vi "Single Bscan - DAQ Trigger.vi"(6 "Frequency":cluster{"Clock, kHz":dbl, "Freq, kHz":dbl}={"Clock, kHz"=935.6, "Freq, kHz"=46.78} {"Clock, kHz" format="%#_13g"}, 7 "# Extra":cluster{"# ARpt_extra":i32, "#Brtn_extra":i32}={"# ARpt_extra"=5, "#Brtn_extra"=40}, 9 "Galvo VPP":cluster{"VPP-X":dbl, "VPP-Y":dbl}={"VPP-X"=5.0, "VPP-Y"=5.0}, 10 "Scan Repeat":cluster{"# A rpt":i32, "# B rpt":i32}={"# A rpt"=1, "# B rpt"=1}, 11 "# Points":cluster{"# Aline":i32, "# B scan":i32}={"# Aline"=500, "# B scan"=500}) -> (2 "Galvo X&Trigger":waveform(dbl)[](graph)=[{"t0"=timestamp(0 s since 1904-01-01), "dt"=1.0, "Y"=array[8820 elements]}, {"t0"=timestamp(0 s since 1904-01-01), "dt"=1.0, "Y"=array[8820 elements]}])   [LabVIEW 2017]
uses:
  <vilib>/Waveform/WDTOps.llb/WDT Append Waveforms DBL.vi
  <vilib>/measure/NI_MABase.lvlib
panel:
  out "# A Rpt Delay":i32
  out "# B rtn":i32
  out "# A repeat":i32
  out "dVX":dbl
  out "S/F":dbl
  out "VPP-Y":dbl
  out "VPP-X":dbl
  out "Clock, kHz":dbl
  out "Freq, kHz":dbl
  out "# A Total":i32
  out "# Aline":i32
  out "# B scan":i32
  out "# B Repeat":i32
  # "Single Bscan - DAQ Trigger"
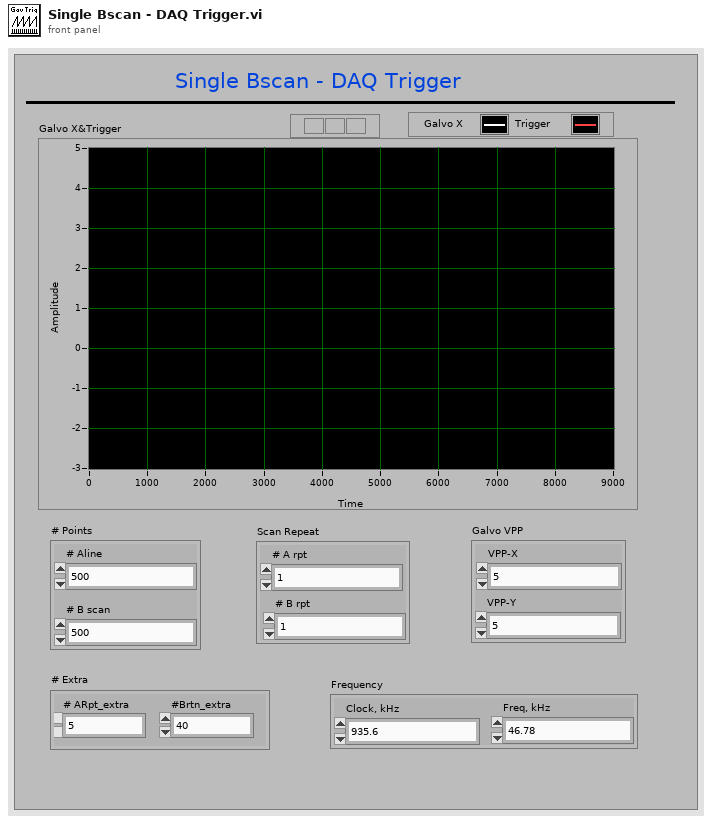
[diagram p1: front panel]
types:
  T1 = enum16{"Sine Wave", "Triangle Wave", "Square Wave", "Sawtooth Wave"}
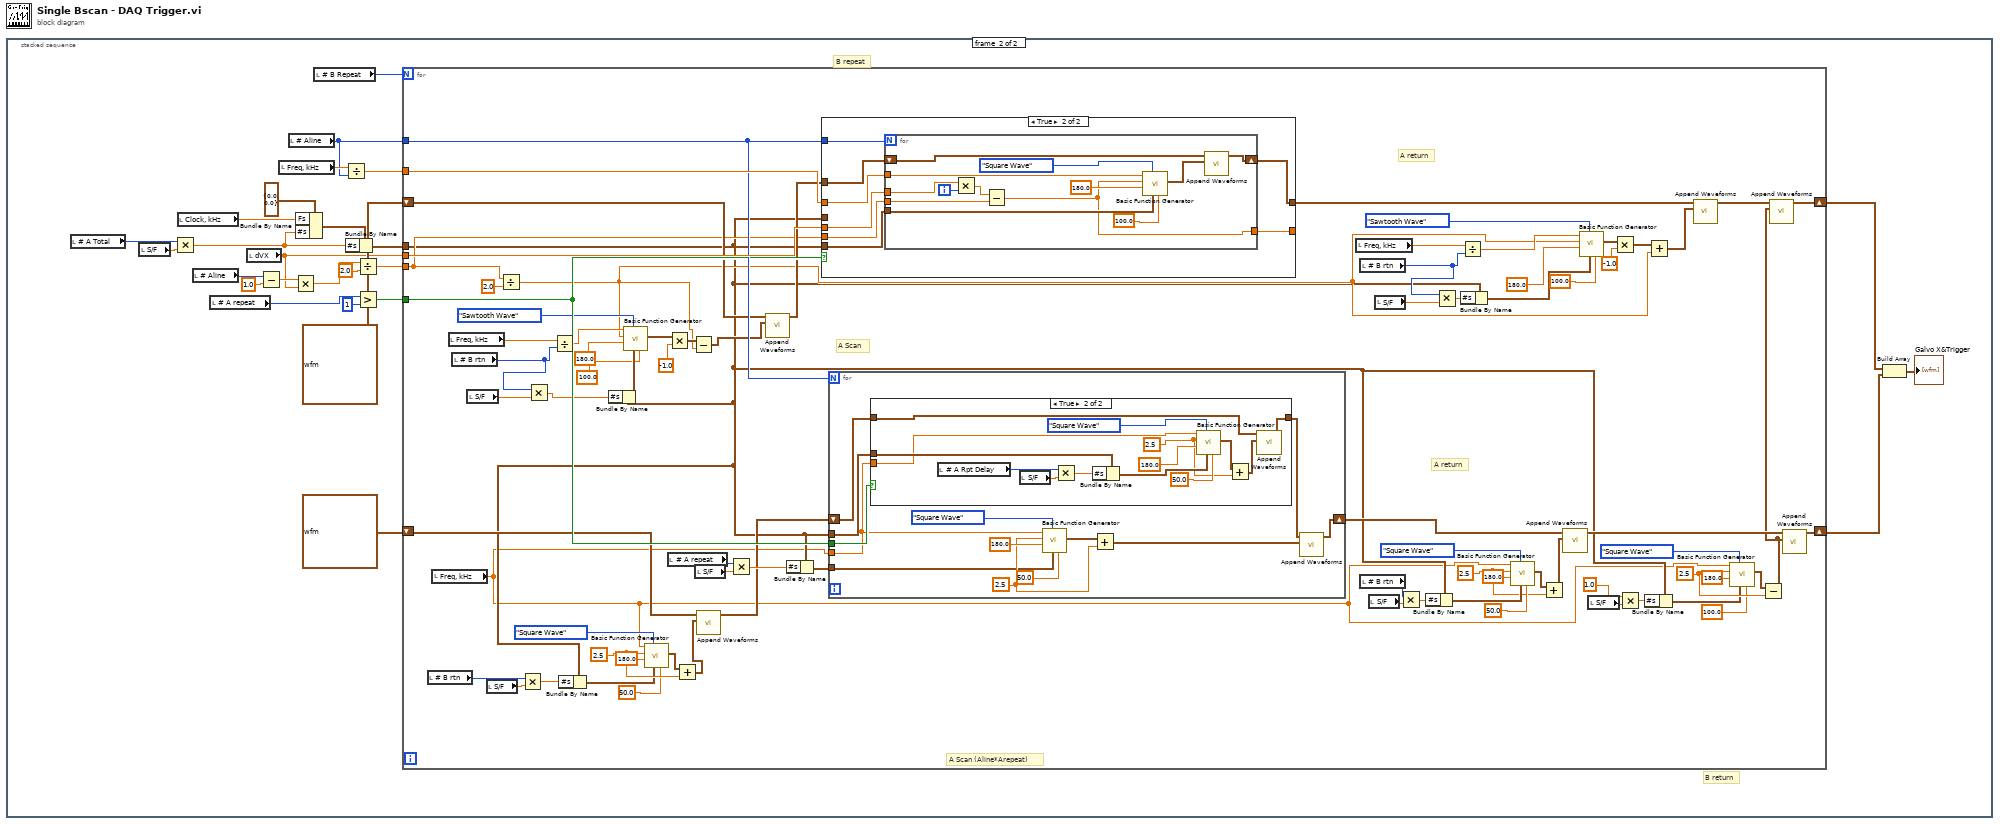
[diagram p0: block diagram]
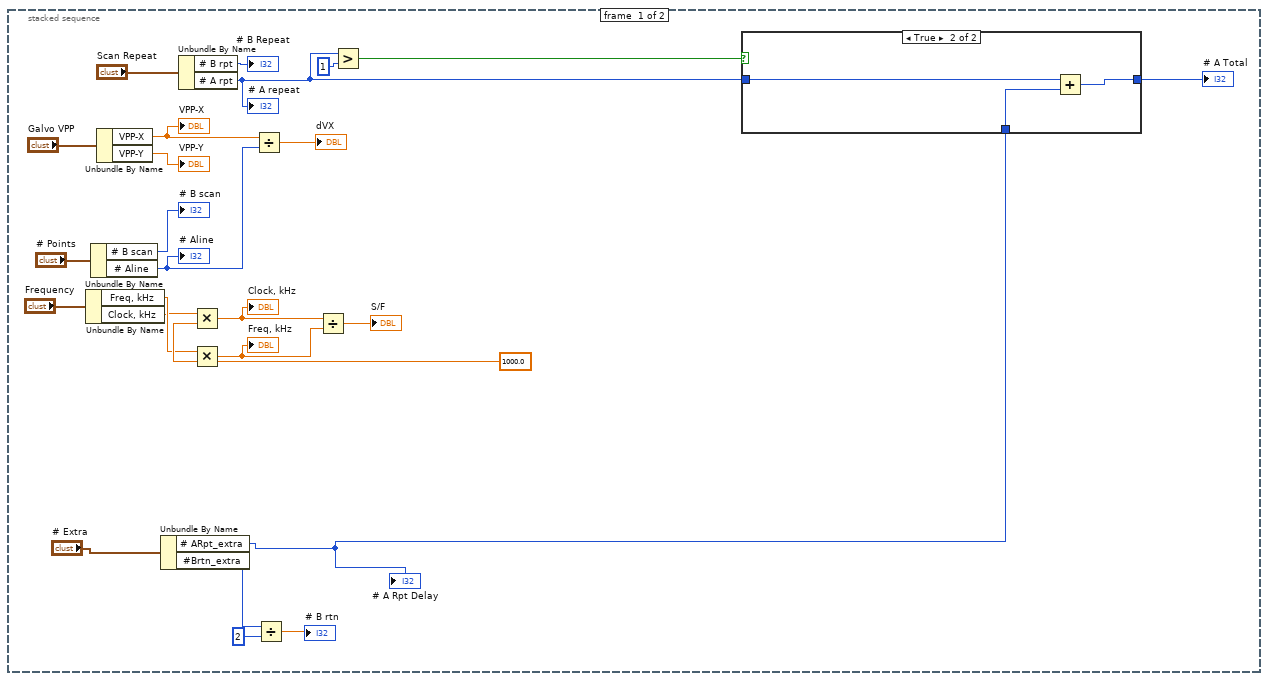
[diagram p2: hidden frame]
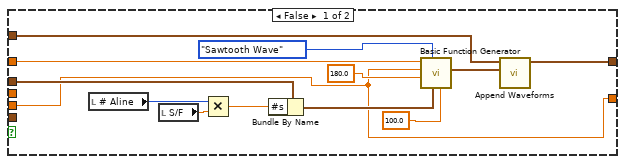
[diagram p5: hidden frame]
diagram:
  n1 = stacked-sequence {
    frame #0 {
      w24 = 1000.0 ("y")
      n2 = Unbundle By Name("Frequency") -> ("Freq, kHz"=w23:dbl, "Clock, kHz"=w19:dbl)
      n3 = Unbundle By Name("# Points") -> ("# B scan"=→"# B scan":i32, "# Aline"=w9:i32)
      "# Aline" <- w9
      n4 = Unbundle By Name("Galvo VPP") -> ("VPP-X"=w8:dbl, "VPP-Y"=→"VPP-Y":dbl)
      "VPP-X" <- w8
      n5 = Unbundle By Name("# Extra") -> ("# ARpt_extra"=w5:i32, "#Brtn_extra"=w4:i32)
      "# A Rpt Delay" <- w5
      n6 = Unbundle By Name("Scan Repeat") -> ("# B rpt"=→"# B Repeat":i32, "# A rpt"=w6:i32)
      "# A repeat" <- w6
      n7 = Multiply(x=w19, y=w24) -> (x*y=w12:dbl)
      "Clock, kHz" <- w12
      n8 = Multiply(x=w23, y=w24) -> (x*y=w11:dbl)
      "Freq, kHz" <- w11
      n9 = Divide(x=w8, y=w9) -> (x/y=→"dVX":dbl)
      n10 = Divide(x=w4, y=2) -> (x/y=→"# B rtn":dbl)
      n11 = Divide(x=w12, y=w11) -> (x/y=→"S/F":dbl)
      n12 = Greater?(x=w6, y=1) -> (0:w20:bool)
      n13 = case shown="True" w20 {
        tunnel: w6 -> [w26 w29]
        tunnel: [w26 w28] -> w22
        tunnel: w5 -> [_ w27]
        frame False {
        }
        frame True {
          n14 = Add(x=w29, y=w27) -> (x+y=w28:i32)
        }
      }
      "# A Total" <- w22
    }
    frame #1 {
      # "B return"
      # "B repeat"
      n15 = local read "# A Total"() -> (w42:i32)
      n16 = local read "S/F"() -> (w41:dbl)
      n17 = Multiply(x=w42, y=w41) -> (x*y=w40:dbl)
      n18 = local read "Clock, kHz"() -> (w43:dbl)
      n19 = local read "# Aline"() -> (w44:i32)
      n20 = local read "# A repeat"() -> (w39:i32)
      n21 = local read "dVX"() -> (w33:dbl)
      n22 = Subtract(x=w44, y=1.0) -> (x-y=w46:dbl)
      n23 = local read "Freq, kHz"() -> (w36:dbl)
      n24 = local read "# Aline"() -> (w35:i32)
      n25 = Multiply(x=w46, y=w33) -> (x*y=w50:dbl)
      n26 = Bundle By Name(cluster=cluster{"Fs":dbl, "#s":dbl} {"Fs"=0.0, "#s"=0.0} ("input cluster"), "Fs"=w43, "#s"=w40) -> (w51:cluster{"Fs":dbl, "#s":dbl})
      n27 = local read "# B Repeat"() -> (w45:i32)
      n28 = Divide(x=w36, y=w35) -> (x/y=w34:dbl)
      n29 = Bundle By Name(cluster=w51, "#s"=w40) -> (w53:cluster{"Fs":dbl, "#s":dbl})
      n30 = Divide(x=w50, y=2.0) -> (x/y=w48:dbl)
      n31 = Greater?(x=w39, y=1) -> (0:w37:bool)
      n32 = for {
        N: w45 -> [_]
        tunnel: w35 -> [w110]
        tunnel: w33 -> [w134]
        tunnel: w53 -> [w61]
        tunnel: w48 -> [w94]
        shift-right: [w58] -> w30
        shift-left: waveform(dbl) {"t0"=timestamp(0 s since 1904-01-01), "dt"=1.0, "Y"=[]} ("waveform out") -> [w98]
        tunnel: w37 -> [w109]
        tunnel: w34 -> [w133]
        shift-right: [w62] -> w31
        shift-left: waveform(dbl) {"t0"=timestamp(0 s since 1904-01-01), "dt"=1.0, "Y"=[]} ("waveform out") -> [w75]
        w70 = 2.5 ("amplitude")
        w84 = 2.5 ("amplitude")
        w85 = 2.5 ("amplitude")
        # "A Scan"
        # "A return"
        # "A Scan (Aline*Arepeat)"
        # "A return"
        n33 = local read "# B rtn"() -> (w79:i32)
        n34 = local read "Freq, kHz"() -> (w60:dbl)
        n35 = local read "Freq, kHz"() -> (w104:dbl)
        n36 = local read "# B rtn"() -> (w107:i32)
        n37 = local read "S/F"() -> (w103:dbl)
        n38 = local read "S/F"() -> (w80:dbl)
        n39 = Divide(x=w94, y=2.0) -> (x/y=w88:dbl)
        n40 = Multiply(x=w79, y=w80) -> (x*y=w81:dbl)
        n41 = Multiply(x=w107, y=w103) -> (x*y=w106:dbl)
        n42 = Divide(x=w104, y=w107) -> (x/y=w105:dbl)
        n43 = Bundle By Name(cluster=w61, "#s"=w81) -> (w76:cluster{"Fs":dbl, "#s":dbl})
        n44 = Bundle By Name(cluster=w61, "#s"=w106) -> (w102:cluster{"Fs":dbl, "#s":dbl})
        n45 = call <vilib>:"Basic Function Generator.vi"("square wave duty cycle (%)"=100.0, "sampling info"=w102, "signal type"=T1."Sawtooth Wave", "phase"=180.0, "amplitude"=w88, "frequency"=w105) -> ("signal out"=w96:waveform(dbl))  [unwired: 3 in, 2 out]
        n46 = call <vilib>:"Basic Function Generator.vi"("square wave duty cycle (%)"=50.0, "sampling info"=w76, "signal type"=T1."Square Wave", "phase"=180.0, "amplitude"=w84, "frequency"=w60) -> ("signal out"=w82:waveform(dbl))  [unwired: 3 in, 2 out]
        n47 = Multiply(x=w96, y=-1.0) -> (x*y=w92:waveform(dbl))
        n48 = local read "# A repeat"() -> (w116:i32)
        n49 = Add(x=w82, y=w84) -> (x+y=w83:waveform(dbl))
        n50 = Subtract(x=w92, y=w88) -> (x-y=w91:waveform(dbl))
        n51 = local read "S/F"() -> (w114:dbl)
        n52 = call-poly <vilib>:"Append Waveforms.vi"("waveform B"=w83, "waveform A"=w75) -> ("waveform out"=w74:waveform(dbl))  [unwired: 8 in, 1 out]
        n53 = Multiply(x=w116, y=w114) -> (x*y=w115:dbl)
        n54 = call-poly <vilib>:"Append Waveforms.vi"("waveform B"=w91, "waveform A"=w98) -> ("waveform out"=w97:waveform(dbl))  [unwired: 8 in, 1 out]
        n55 = Bundle By Name(cluster=w61, "#s"=w115) -> (w119:cluster{"Fs":dbl, "#s":dbl})
        n56 = case shown="True" w109 {
          tunnel: w97 -> [w164 w183]
          tunnel: w110 -> [_ w182]
          tunnel: w134 -> [_ w181]
          tunnel: w61 -> [_ w180]
          tunnel: w94 -> [w163 w179]
          tunnel: [w165 w178] -> w126
          tunnel: [w163 w177] -> _
          tunnel: w133 -> [w172 w176]
          tunnel: w61 -> [w170 _]
          frame False {
            n57 = local read "# Aline"() -> (w169:i32)
            n58 = local read "S/F"() -> (w168:dbl)
            n59 = Multiply(x=w169, y=w168) -> (x*y=w167:dbl)
            n60 = Bundle By Name(cluster=w170, "#s"=w167) -> (w171:cluster{"Fs":dbl, "#s":dbl})
            n61 = call <vilib>:"Basic Function Generator.vi"("square wave duty cycle (%)"=100.0, "sampling info"=w171, "signal type"=T1."Sawtooth Wave", "phase"=180.0, "amplitude"=w163, "frequency"=w172) -> ("signal out"=w166:waveform(dbl))  [unwired: 3 in, 2 out]
            n62 = call-poly <vilib>:"Append Waveforms.vi"("waveform B"=w166, "waveform A"=w164) -> ("waveform out"=w165:waveform(dbl))  [unwired: 8 in, 1 out]
          }
          frame True {
            n63 = for {
              N: w182 -> [_]
              tunnel: w176 -> [w190]
              tunnel: w180 -> [w194]
              tunnel: w181 -> [w192]
              shift-right: [w189] -> w178
              shift-left: w183 -> [w188]
              tunnel: w179 -> [w186]
              tunnel: [w185] -> w177
              i -> [w191]
              n64 = Multiply(x=w192, y=w191) -> (x*y=w187:dbl)
              n65 = Subtract(x=w187, y=w186) -> (x-y=w185:dbl)
              n66 = call <vilib>:"Basic Function Generator.vi"("square wave duty cycle (%)"=100.0, "sampling info"=w194, "signal type"=T1."Square Wave" ("signal type B"), "phase"=180.0, "amplitude"=w185, "frequency"=w190) -> ("signal out"=w195:waveform(dbl))  [unwired: 3 in, 2 out]
              n67 = call-poly <vilib>:"Append Waveforms.vi"("waveform B"=w195, "waveform A"=w188) -> ("waveform out"=w189:waveform(dbl))  [unwired: 8 in, 1 out]
            }
          }
        }
        n68 = for {
          N: w110 -> [_]
          tunnel: w119 -> [w140]
          tunnel: w61 -> [w139]
          tunnel: w109 -> [w138]
          tunnel: w60 -> [w137]
          shift-right: [w147] -> w121
          shift-left: w74 -> [w135]
          w141 = 2.5 ("amplitude")
          n69 = case shown="True" w138 {
            tunnel: w139 -> [_ w160]
            tunnel: w137 -> [_ w158]
            tunnel: [w148 w153] -> w136
            tunnel: w135 -> [w148 w154]
            frame False {
            }
            frame True {
              w149 = 2.5 ("amplitude")
              n70 = local read "# A Rpt Delay"() -> (w155:i32)
              n71 = local read "S/F"() -> (w156:dbl)
              n72 = Multiply(x=w155, y=w156) -> (x*y=w162:dbl)
              n73 = Bundle By Name(cluster=w160, "#s"=w162) -> (w161:cluster{"Fs":dbl, "#s":dbl})
              n74 = call <vilib>:"Basic Function Generator.vi"("square wave duty cycle (%)"=50.0, "sampling info"=w161, "signal type"=T1."Square Wave", "phase"=180.0, "amplitude"=w149, "frequency"=w158) -> ("signal out"=w152:waveform(dbl))  [unwired: 3 in, 2 out]
              n75 = Add(x=w152, y=w149) -> (x+y=w150:waveform(dbl))
              n76 = call-poly <vilib>:"Append Waveforms.vi"("waveform B"=w150, "waveform A"=w154) -> ("waveform out"=w153:waveform(dbl))  [unwired: 8 in, 1 out]
            }
          }
          n77 = call <vilib>:"Basic Function Generator.vi"("square wave duty cycle (%)"=50.0, "sampling info"=w140, "signal type"=T1."Square Wave" ("signal type B"), "phase"=180.0, "amplitude"=w141, "frequency"=w137) -> ("signal out"=w143:waveform(dbl))  [unwired: 3 in, 2 out]
          n78 = Add(x=w143, y=w141) -> (x+y=w142:waveform(dbl))
          n79 = call-poly <vilib>:"Append Waveforms.vi"("waveform B"=w142, "waveform A"=w136) -> ("waveform out"=w147:waveform(dbl))  [unwired: 8 in, 1 out]
        }
        n80 = local read "Freq, kHz"() -> (w125:dbl)
        n81 = local read "# B rtn"() -> (w108:i32)
        n82 = local read "# B rtn"() -> (w113:i32)
        n83 = local read "S/F"() -> (w112:dbl)
        n84 = local read "S/F"() -> (w128:dbl)
        n85 = Multiply(x=w113, y=w112) -> (x*y=w111:dbl)
        n86 = Bundle By Name(cluster=w61, "#s"=w111) -> (w120:cluster{"Fs":dbl, "#s":dbl})
        n87 = Multiply(x=w108, y=w128) -> (x*y=w123:dbl)
        n88 = Divide(x=w125, y=w108) -> (x/y=w124:dbl)
        n89 = Bundle By Name(cluster=w61, "#s"=w123) -> (w129:cluster{"Fs":dbl, "#s":dbl})
        n90 = call <vilib>:"Basic Function Generator.vi"("square wave duty cycle (%)"=50.0, "sampling info"=w120, "signal type"=T1."Square Wave", "phase"=180.0, "amplitude"=w85, "frequency"=w60) -> ("signal out"=w87:waveform(dbl))  [unwired: 3 in, 2 out]
        n91 = Add(x=w87, y=w85) -> (x+y=w86:waveform(dbl))
        n92 = call-poly <vilib>:"Append Waveforms.vi"("waveform B"=w86, "waveform A"=w121) -> ("waveform out"=w63:waveform(dbl))  [unwired: 8 in, 1 out]
        n93 = call <vilib>:"Basic Function Generator.vi"("square wave duty cycle (%)"=100.0, "sampling info"=w129, "signal type"=T1."Sawtooth Wave", "phase"=180.0, "amplitude"=w88, "frequency"=w124) -> ("signal out"=w122:waveform(dbl))  [unwired: 3 in, 2 out]
        n94 = local read "S/F"() -> (w67:dbl)
        n95 = Multiply(x=w122, y=-1.0) -> (x*y=w90:waveform(dbl))
        n96 = Multiply(x=1.0, y=w67) -> (x*y=w68:dbl)
        n97 = Bundle By Name(cluster=w61, "#s"=w68) -> (w64:cluster{"Fs":dbl, "#s":dbl})
        n98 = Add(x=w90, y=w88) -> (x+y=w89:waveform(dbl))
        n99 = call-poly <vilib>:"Append Waveforms.vi"("waveform B"=w89, "waveform A"=w126) -> ("waveform out"=w57:waveform(dbl))  [unwired: 8 in, 1 out]
        n100 = call <vilib>:"Basic Function Generator.vi"("square wave duty cycle (%)"=100.0, "sampling info"=w64, "signal type"=T1."Square Wave", "phase"=180.0, "amplitude"=w70, "frequency"=w60) -> ("signal out"=w69:waveform(dbl))  [unwired: 3 in, 2 out]
        n101 = Subtract(x=w69, y=w70) -> (x-y=w56:waveform(dbl))
        n102 = call-poly <vilib>:"Append Waveforms.vi"("waveform B"=w56, "waveform A"=w57) -> ("waveform out"=w58:waveform(dbl))  [unwired: 8 in, 1 out]
        n103 = call-poly <vilib>:"Append Waveforms.vi"("waveform B"=w56, "waveform A"=w63) -> ("waveform out"=w62:waveform(dbl))  [unwired: 8 in, 1 out]
      }
      n104 = Build Array(w30, w31) -> (→"Galvo X&Trigger":waveform(dbl)[])
    }
  }
